vi "example_2_2_b.vi"() -> ()   [LabVIEW 2018]
panel:
  out "Result":dbl format="%.2f"
  in  "Number 2":dbl format="%.2f"
  in  "Number 1":dbl format="%.2f"
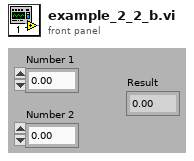
[diagram p1: front panel]
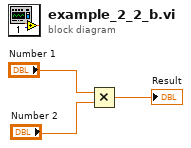
[diagram p0: block diagram]
diagram:
  n1 = Multiply(x="Number 1", y="Number 2") -> (x*y=→"Result":dbl)
